vi "traitement_son.vi"(6 "Nb de valeurs par moyenne":i32, 8 "Erreur IN TRAITEMENT":errorcluster, 9 "Entrée file TRAITEMENT":refnum<queue>, 10 "Erreur IN ACQ":errorcluster, 11 "Entrée file ACQ":refnum<queue>) -> (0 "Erreur OUT TRAITEMENT":errorcluster, 1 "Sortie file TRAITEMENT":refnum<queue>, 2 "Erreur OUT ACQ":errorcluster, 3 "Sortie file ACQ":refnum<queue>)   [LabVIEW 2017]
doc: "Sous-vi gérant le traitement du son : filtrage, DSP, plusieurs moyennes sur plage de fréquences audibles renvoyées dans une file."
uses:
  <vilib>/Analysis/4window.llb/windowTd.ctl
  <vilib>/Analysis/3filter.llb/Filter Structure Type.ctl
  variable_stop_globale.vi
  <vilib>/measure/macond.llb/IIR Filter for N Chan.vi
  <vilib>/measure/maspectr.llb/FFT Power Spectrum and PSD for N Chan.vi
  <vilib>/measure/NI_MAPro.lvlib
  <vilib>/Analysis/NI_AALPro.lvlib
  <vilib>/Analysis/NI_AALBase.lvlib
panel:
  out "Son reçu":waveform(dbl)[](graph)
  out "Power Spectrum / PSD":cluster{"f0":dbl, "df":dbl, "magnitude":dbl[]}[](array[cluster]) caption="Spectre de puissance / DSP" {"magnitude" format="%.2p"; "f0" format="%.2p"; "df" format="%.2p"}
  out "DSP":cluster{"f0":dbl, "df":dbl, "magnitude":dbl[]}[](graph)
  out "Tableau":dbl[](array[numeric])
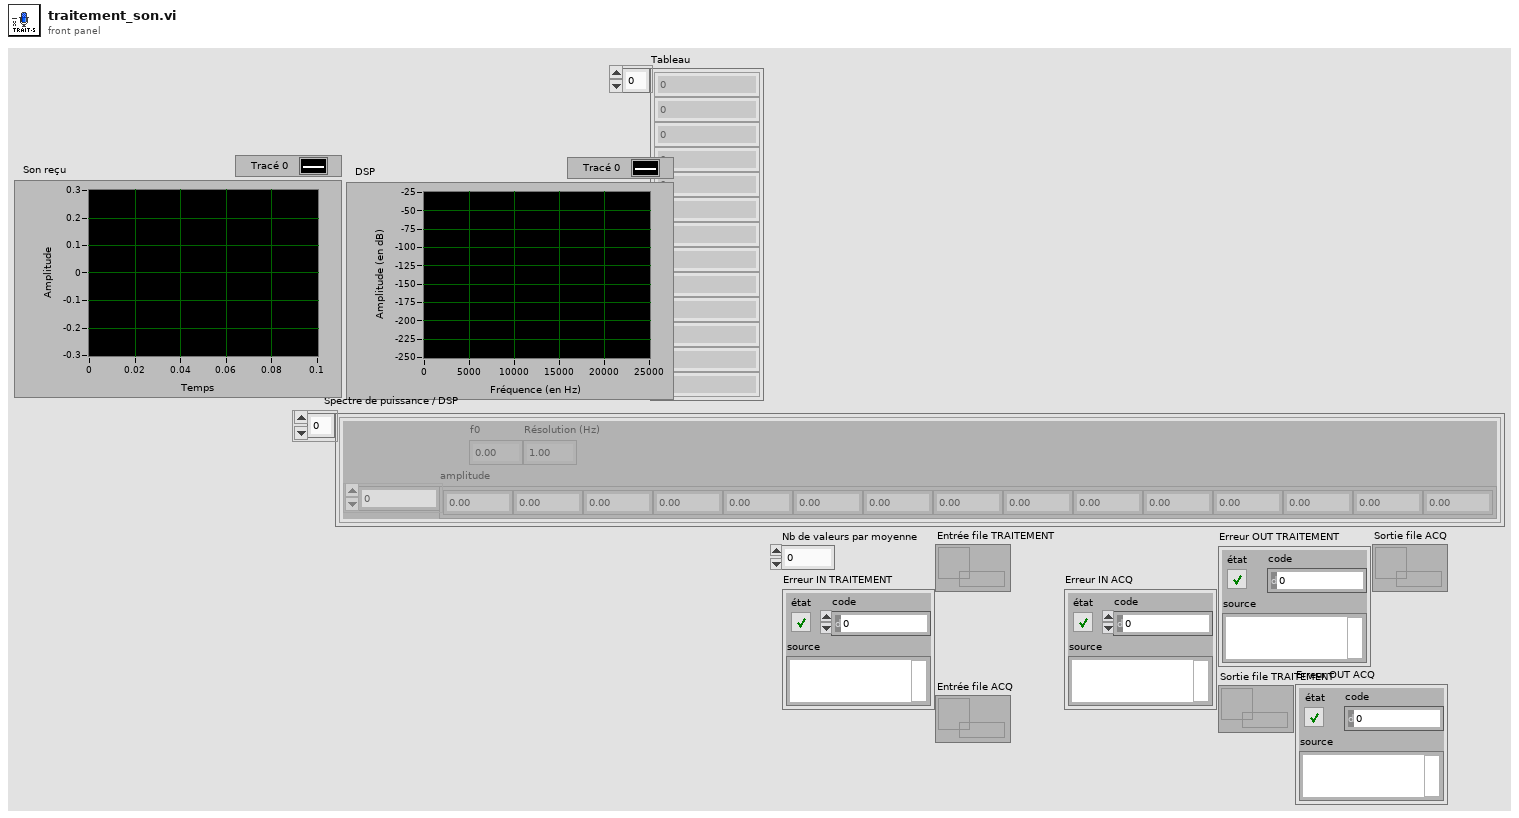
[diagram p1: front panel]
types:
  T1 = typedef "NI_AALBase.lvlib/Filter Structure Type.ctl" = u16
  T2 = typedef "NI_AALPro.lvlib/windowTd.ctl" = u32
  T3 = cluster{"Topology":enum16{"Off", "Butterworth", "Chebyshev", "Inverse Chebyshev", "Elliptic", "Bessel"}, "Type":enum16{"Lowpass", "Highpass", "Bandpass", "Bandstop"}, "Order":i32, "Lower Fc":dbl, "Upper Fc":dbl, "PB Ripple":dbl, "SB Attenuation":dbl}
  T4 = cluster{"Power Spectrum / PSD[0]":cluster{"f0":dbl, "df":dbl, "magnitude":dbl[]}, "Power Spectrum / PSD[1]":cluster{"f0":dbl, "df":dbl, "magnitude":dbl[]}, "Power Spectrum / PSD[2]":cluster{"f0":dbl, "df":dbl, "magnitude":dbl[]}, "Power Spectrum / PSD[3]":cluster{"f0":dbl, "df":dbl, "magnitude":dbl[]}, "Power Spectrum / PSD[4]":cluster{"f0":dbl, "df":dbl, "magnitude":dbl[]}, "Power Spectrum / PSD[5]":cluster{"f0":dbl, "df":dbl, "magnitude":dbl[]}, "Power Spectrum / PSD[6]":cluster{"f0":dbl, "df":dbl, "magnitude":dbl[]}, "Power Spectrum / PSD[7]":cluster{"f0":dbl, "df":dbl, "magnitude":dbl[]}, "Power Spectrum / PSD[8]":cluster{"f0":dbl, "df":dbl, "magnitude":dbl[]}}
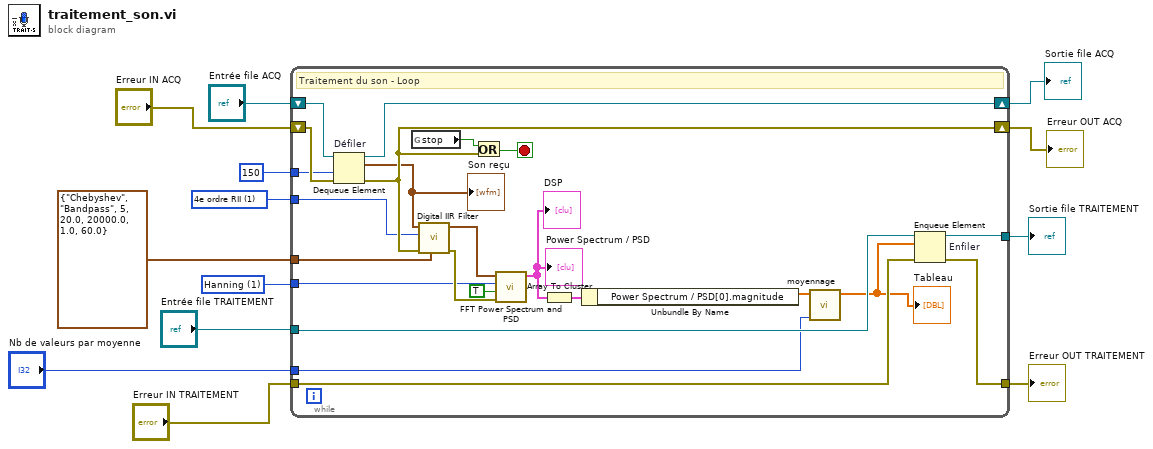
[diagram p0: block diagram]
diagram:
  w10 = T1 1 items=["2e ordre RII"=0, "4e ordre RII"=1, "Sélection automatique"=10] ("filter structure option")
  w2 = T2 1 items=["Rectangle"=0, "Hanning"=1, "Hamming"=2, "Blackman-Harris"=3, "Blackman exacte"=4, "Blackman"=5, "Profil plat"=6, "B-Harris 4 termes "=7, "B-Harris 7 termes"=8, "Lobe latéral bas"=9, "Blackman Nuttall"=11, "Triangle"=30, "Bartlett-Hanning"=31, "Bohman"=32, "Parzen"=33, "Welch"=34, "Kaiser"=60, "Dolph-Tchebychev"=61, "Gaussienne"=62] ("window")
  n1 = while "Boucle While" {
    shift-right: [w30] -> w4
    shift-left: "Erreur IN ACQ" -> [w35]
    shift-right: [w34] -> w3
    shift-left: "Entrée file ACQ" -> [w36]
    tunnel: 150 ("timeout en ms") -> [w33]
    tunnel: w10 -> [w16]
    tunnel: T3 {"Topology"=enum."Chebyshev", "Type"=enum."Bandpass", "Order"=5, "Lower Fc"=20.0, "Upper Fc"=20000.0, "PB Ripple"=1.0, "SB Attenuation"=60.0} ("IIR filter specifications") -> [w28]
    tunnel: w2 -> [w27]
    tunnel: "Entrée file TRAITEMENT" -> [w20]
    tunnel: [w21] -> w5
    tunnel: [w17] -> w6
    tunnel: "Erreur IN TRAITEMENT" -> [w22]
    tunnel: "Nb de valeurs par moyenne" -> [w15]
    stop <- w32 stop-if-true
    # "Traitement du son - Loop"
    n2 = Dequeue Element "Défiler"(queue=w36, timeout in ms (-1)=w33, error in (no error)=w35) -> (queue out=w34:refnum<queue>, element=w19:waveform(dbl)[], error out=w30:errorcluster)  [unwired: 1 out]
    "Son reçu" <- w19
    n3 = global read "variable_stop_globale.vi" "stop"() -> (w14:bool)
    n4 = call-poly <vilib>:"Digital IIR Filter.vi"("IIR filter specifications"=w28, "error in (no error)"=w30, "filter structure option"=w16, "signal(s) in"=w19) -> ("error out"=w29:errorcluster, "signal(s) out"=w31:waveform(dbl)[])  [unwired: 5 in, 1 out]
    n5 = Or(x=w14, y=w30) -> (x .or. y?=w32:bool)
    n6 = call-poly <vilib>:"FFT Power Spectrum and PSD.vi"("error in (no error)"=w29, "dB On (F)"=TRUE, "window"=w27, "time signals"=w31) -> ("Power Spectrum / PSD"=w24:cluster{"f0":dbl, "df":dbl, "magnitude":dbl[]}[])  [unwired: 4 in, 3 out]
    "Power Spectrum / PSD" <- w24
    "DSP" <- w24
    n7 = Array To Cluster(array=w24) -> (cluster=w25:T4)
    n8 = Unbundle By Name(w25) -> ("Power Spectrum / PSD[0].magnitude"=w23:dbl[])
    n9 = call "moyennage.vi"("Nb de valeurs par moyenne"=w15, "DSP Amplitude"=w23) -> ("DSP Amplitude Moyenné"=w18:dbl[])  [unwired: 9 in]
    "Tableau" <- w18
    n10 = Enqueue Element "Enfiler"(queue=w20, element=w18, error in (no error)=w22) -> (queue out=w21:refnum<queue>, error out=w17:errorcluster)  [unwired: 1 in, 1 out]
  }
  "Erreur OUT TRAITEMENT" <- w6
  "Sortie file TRAITEMENT" <- w5
  "Erreur OUT ACQ" <- w4
  "Sortie file ACQ" <- w3
